vi "AM Initialize Hardware References.vi"(8 "error in (no error)":errorcluster, 10 "Message Data":variant, 11 "Hardware Resources in":T1) -> (0 "error out":errorcluster, 3 "Hardware Resources out":T1)   [LabVIEW 2020, in "Motion.lvlib"]
doc: "Initialize the hardware references."
uses:
  Motion.lvlib
  AM Configuration.ctl
  support/Message Queue/Message Cluster.ctl
  support/Message Queue/Message Queue.lvlib
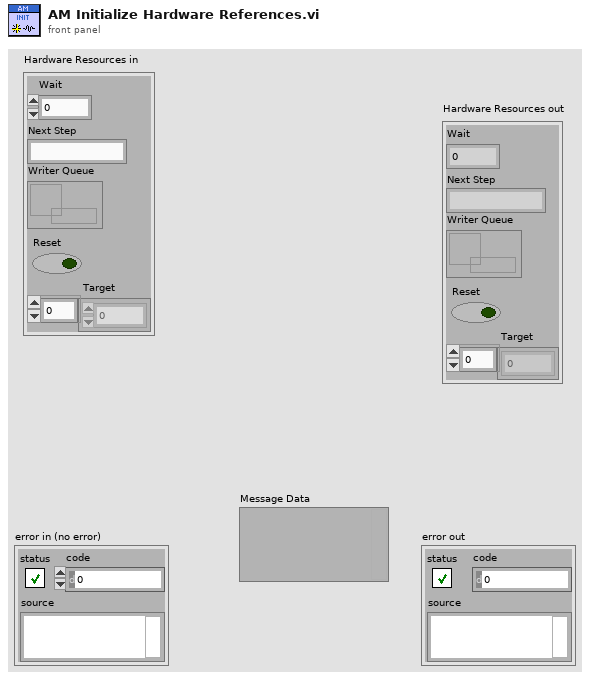
[diagram p1: front panel]
types:
  T1 = typedef "Motion.lvlib/AM Configuration.ctl" = cluster{"Wait":dbl, "Next Step":string, "Writer Queue":refnum<queue>, "Reset":bool, "Target":dbl[]}
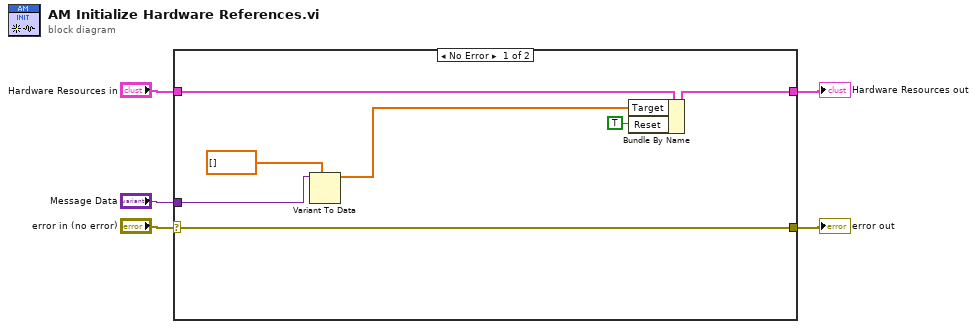
[diagram p0: block diagram]
diagram:
  n1 = case shown="No Error" "error in (no error)" {
    selector: "error in (no error)" -> [w11 w13]
    tunnel: [w11 w13] -> w4
    tunnel: "Hardware Resources in" -> [w12 w14]
    tunnel: [w9 w14] -> w1
    tunnel: "Message Data" -> [w10 _]
    frame No Error {
      n2 = Variant To Data(type=dbl[] [] ("Current SP"), Variant=w10) -> (data=w8:dbl[])  [unwired: 1 in, 1 out]
      n3 = Bundle By Name(cluster=w12, "Target"=w8, "Reset"=TRUE) -> (w9:T1)
    }
    frame Error {
    }
  }
  "Hardware Resources out" <- w1
  "error out" <- w4
